vi "niRFUtil MT UTIL Generate Bits Pattern.vi"(0 "Total Bits":i32, 2 "Reset? (T)":bool=TRUE, 5 "User Base Bit Pattern":T1 min=0) -> (4 "Output Bit Stream":T1 min=0)   [LabVIEW 2015, in "niRFUtil.lvlib"]
doc: "Generates a bit sequence using the specified pattern. The pattern is replicated until you reach Total Bits."
uses:
  niRFUtil.lvlib
  Includes/niRFUtil INC Bit Array.ctl
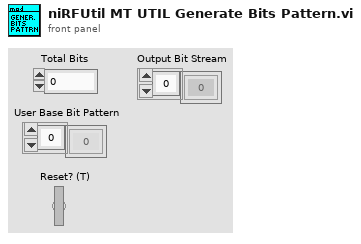
[diagram p1: front panel]
types:
  T1 = typedef "niRFUtil.lvlib/niRFUtil INC Bit Array.ctl" = i8[]
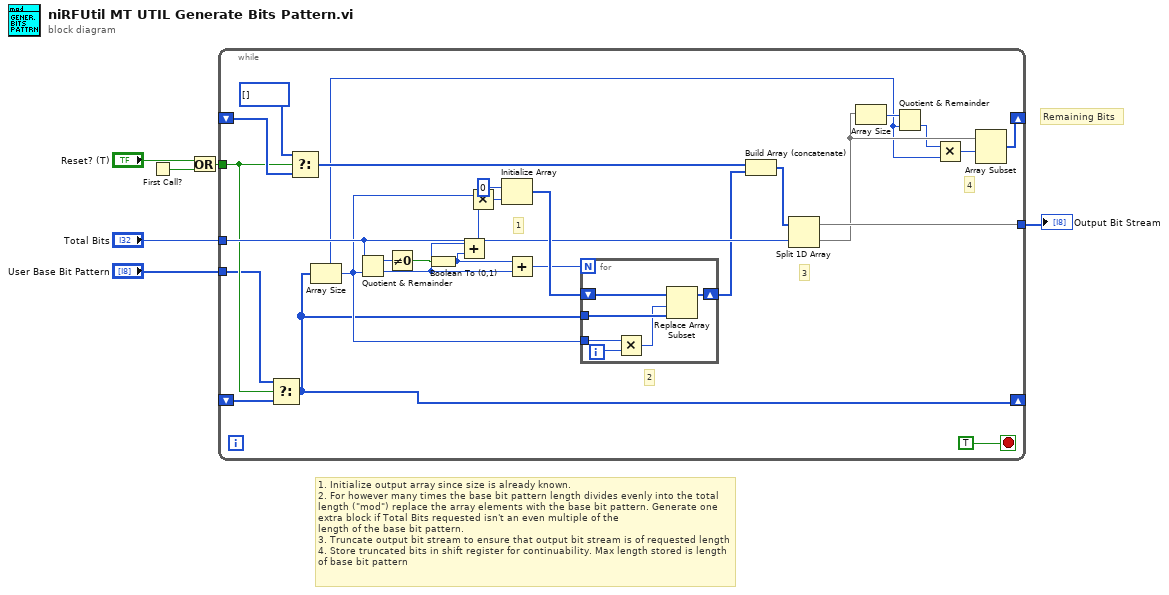
[diagram p0: block diagram]
diagram:
  # "Remaining Bits"
  # "1. Initialize output array since size is already known.\n2. For however many times the base bit pattern length divides evenly into the total length (\"mod\") replace the array elements with the base bit pattern. Generate one extra block if Total Bits requested isn't an even multiple of the\nlength of the base bit pattern.\n3. Truncate output bit stream to ensure that output bit stream is of requested length\n4. Store truncated bits in shift register for continuability. Max length stored is length of base bit pattern"
  n1 = First Call?() -> (First Call?: T/F=w3:bool)
  n2 = Or(x="Reset? (T)", y=w3) -> (x .or. y?=w1:bool)
  n3 = while {
    tunnel: "User Base Bit Pattern" -> [w8]
    tunnel: "Total Bits" -> [w29]
    tunnel: [w28] -> w4
    shift-right: [w15] -> _
    shift-left: _ -> [w27]
    tunnel: w1 -> [w9]
    shift-right: [w7] -> _
    shift-left: _ -> [w10]
    stop <- TRUE stop-if-true
    # "4"
    # "1"
    # "2"
    # "3"
    n4 = Select(t=w8, s=w9, f=w10) -> (s? t:f=w7:T1)
    n5 = Select(t=i8[] [], s=w9, f=w27) -> (s? t:f=w24:i8[])
    n6 = Array Size(array=w7) -> (size(s)=w11:i32)
    n7 = Quotient & Remainder(x=w29, y=w11) -> (x-y*floor(x/y)=w22:i32, floor(x/y)=w17:i32)
    n8 = Not Equal To 0?(x=w22) -> (x != 0?=w30:bool)
    n9 = Boolean To (0,1)(Boolean=w30) -> (0, 1=w21:i16)
    n10 = Add(x=w17, y=w21) -> (x+y=w20:i32)
    n11 = Multiply(x=w11, y=w20) -> (x*y=w19:i32)
    n12 = Initialize Array(i8 0, w19) -> (w33:i8[])
    n13 = Add(x=w21, y=w17) -> (x+y=w31:i32)
    n14 = for {
      N: w31 -> [_]
      shift-right: [w38] -> w23
      shift-left: w33 -> [w39]
      tunnel: w7 -> [w37]
      tunnel: w11 -> [w35]
      i -> [w36]
      n15 = Multiply(x=w35, y=w36) -> (x*y=w34:i32)
      n16 = Replace Array Subset(array=w39, new element=w37, index=w34) -> (w38:i8[])
    }
    n17 = Build Array (concatenate)(w24, w23) -> (w18:i8[])
    n18 = Split 1D Array(array=w18, index=w29) -> (first subarray=w28:i8[], second subarray=w16:i8[])
    n19 = Array Size(array=w16) -> (size(s)=w13:i32)
    n20 = Quotient & Remainder(x=w13, y=w11) -> (floor(x/y)=w14:i32)  [unwired: 1 out]
    n21 = Multiply(x=w14, y=w11) -> (x*y=w12:i32)
    n22 = Array Subset(array=w16, index=w12) -> (w15:i8[])  [unwired: 1 in]
  }
  "Output Bit Stream" <- w4
